vi "Compute Image ROI Statistics.vi"(6 "ROI Characteristics Selection":T1={"Area (pixels)"=TRUE, "% of Image"=TRUE, "Total Intensity"=TRUE, "Mean Intensity"=TRUE, "Median Intensity"=TRUE, "Mode Intensity"=TRUE, "Intensity Standard Deviation"=TRUE, "Min Intensity"=TRUE, "Max Intensity"=TRUE, "Mean SNR"=TRUE, "Median SNR"=TRUE, "Mode SNR"=TRUE, "SNR Standard Deviation"=TRUE, "Max SNR"=TRUE, "Min SNR"=TRUE, "# Rejected Pixels (NaN, Inf)"=TRUE, "# Negative Pixels"=TRUE, "Long Axis Length"=FALSE, "Short Axis Length"=FALSE, "Aspect Ratio"=FALSE}, 8 "error in (no error)":errorcluster, 9 "ROIs":T3(array[cluster]), 10 "ROI Mask Refnum":T4, 11 "Image Refnum":T4) -> (0 "error out":errorcluster, 1 "ROI Characteristics String":string, 3 "ROI Characteristics":T2[](array[typedef]))   [LabVIEW 2021, in "Image.lvlib"]
doc: "<B>Image Refnum</B> is the image to be analyzed.\n\n<B>ROI Mask Refnum</B> is the image used to store the mask image corresponding to the ROI (same type as source image). If no image is provided, a temporary one is c reated (and destroyed after use).\n\n<B>ROI</B> is the ROI descriptor."
uses:
  Image.lvlib
  <vilib>/vision/Image Controls.llb/IMAQ Image.ctl
  Image ROI Statistics.ctl
  Image ROI Statistics Selection.ctl
  <vilib>/vision/NI_Vision_Development_Module.lvlib
  Error/Error.lvlib
  Variant/Variant.lvlib
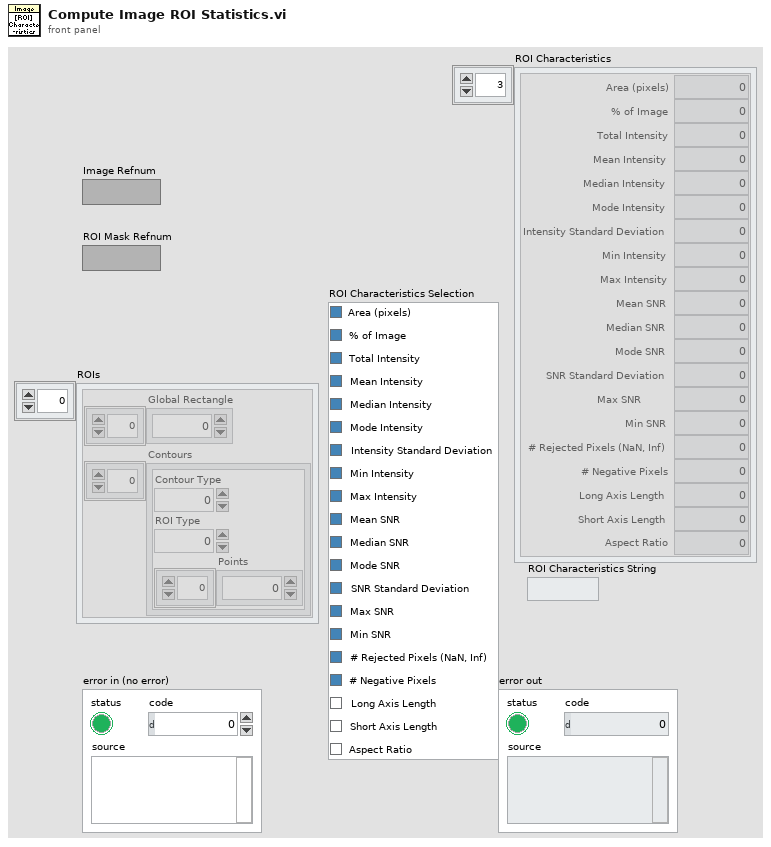
[diagram p1: front panel]
types:
  T1 = typedef "Image.lvlib/Image ROI Statistics Selection.ctl" = cluster{"Area (pixels)":bool, "% of Image":bool, "Total Intensity":bool, "Mean Intensity":bool, "Median Intensity":bool, "Mode Intensity":bool, "Intensity Standard Deviation":bool, "Min Intensity":bool, "Max Intensity":bool, "Mean SNR":bool, "Median SNR":bool, "Mode SNR":bool, "SNR Standard Deviation":bool, "Max SNR":bool, "Min SNR":bool, "# Rejected Pixels (NaN, Inf)":bool, "# Negative Pixels":bool, "Long Axis Length":bool, "Short Axis Length":bool, "Aspect Ratio":bool}
  T2 = typedef "Image.lvlib/Image ROI Statistics.ctl" = cluster{"Area (pixels)":dbl, "% of Image":dbl, "Total Intensity":dbl, "Mean Intensity":dbl, "Median Intensity":dbl, "Mode Intensity":dbl, "Intensity Standard Deviation":dbl, "Min Intensity":dbl, "Max Intensity":dbl, "Mean SNR":dbl, "Median SNR":dbl, "Mode SNR":dbl, "SNR Standard Deviation":dbl, "Max SNR":dbl, "Min SNR":dbl, "# Rejected Pixels (NaN, Inf)":dbl, "# Negative Pixels":dbl, "Long Axis Length":dbl, "Short Axis Length":dbl, "Aspect Ratio":dbl}
  T3 = cluster{"Global Rectangle":i32[], "Contours":cluster{"Contour Type":u32, "ROI Type":u32, "Points":i32[]}[]}[]
  T4 = typedef "IMAQ Image.ctl" = refnum<image>
  T5 = typedef "Image Type" = u32
  T6 = cluster{"Global Rectangle":i32[], "Contours":cluster{"Contour Type":u32, "ROI Type":u32, "Points":i32[]}[]}
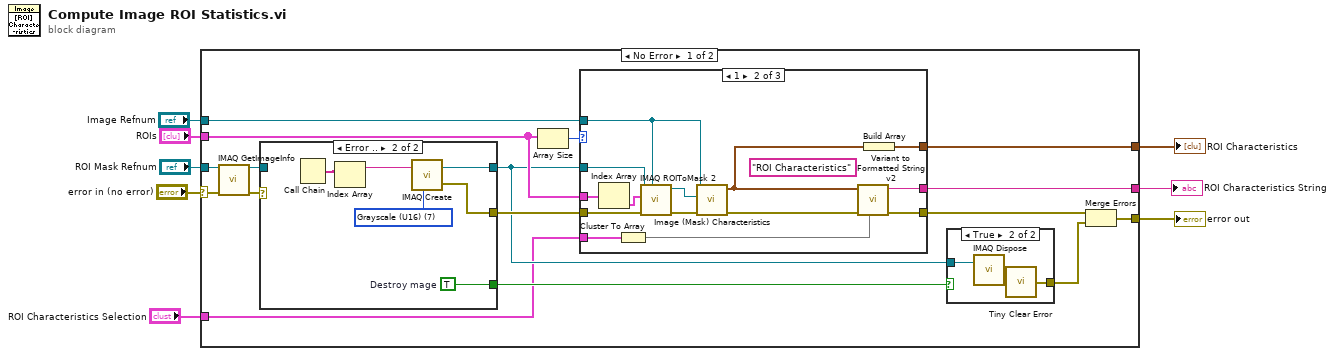
[diagram p0: block diagram]
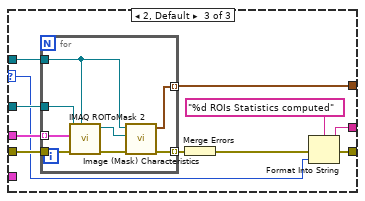
[diagram p4: hidden frame]
diagram:
  n1 = case shown="No Error" "error in (no error)" {
    selector: "error in (no error)" -> [w20 w69]
    tunnel: "Image Refnum" -> [w23 _]
    tunnel: [w22 _] -> w7
    tunnel: [w21 _] -> w6
    tunnel: [w11 w69] -> w5
    tunnel: "ROIs" -> [w16 _]
    tunnel: "ROI Mask Refnum" -> [w18 _]
    tunnel: "ROI Characteristics Selection" -> [w9 _]
    frame No Error {
      n2 = call "IMAQ GetImageInfo"("error in (no error)"=w20, "Image"=w18) -> ("error out"=w19:errorcluster)  [unwired: 2 in, 7 out]
      n3 = case shown="Error .." w19 {
        selector: w19 -> [w62 _]
        tunnel: [w62 w68] -> w17
        tunnel: w18 -> [w61 _]
        tunnel: [w61 w67] -> w13
        tunnel: [_ w63] -> w14
        frame No Error {
        }
        frame Error {
          w66 = T5 7 items=["Grayscale (U8)", "Grayscale (I16)", "Grayscale (SGL)", "Complex (CSG)", "RGB (U32)", "HSL (U32)", "RGB (U64)", "Grayscale (U16)"] ("Image Type")
          w63 = TRUE  # Destroy mage
          n4 = Call Chain() -> (call chain=w65:string[])
          n5 = Index Array(array=w65) -> (element=w64:string)  [unwired: 1 in]
          n6 = call "IMAQ Create"("Image Name"=w64, "Image Type"=w66) -> ("New Image"=w67:T4, "error out"=w68:errorcluster)  [unwired: 3 in]
        }
      }
      n7 = Array Size(array=w16) -> (size(s)=w15:i32)
      n8 = case shown="1" w15 {
        selector: w15 -> [_ _ w42]
        tunnel: w23 -> [_ w41 w52]
        tunnel: [_ w30 w51] -> w22
        tunnel: [_ w39 w44] -> w21
        tunnel: [w27 w38 w45] -> w10
        tunnel: w13 -> [_ w31 w49]
        tunnel: w17 -> [w27 w35 w50]
        tunnel: w16 -> [_ w34 w47]
        tunnel: w9 -> [_ w29 _]
        frame 0 {
        }
        frame 1 {
          (unwired) "ROI Characteristics" ("Label")
          n9 = Index Array(array=w34) -> (element=w33:T6)  [unwired: 1 in]
          n10 = Cluster To Array(cluster=w29) -> (array=w28:bool[])
          n11 = call "IMAQ ROIToMask 2"("Image Model"=w41, "error in (no error)"=w35, "ROI Descriptor"=w33, "Image"=w31) -> ("error out"=w37:errorcluster, "Image Out"=w36:T4)  [unwired: 5 in, 1 out]
          n12 = call "Image (Mask) Characteristics.vi"("error in (no error)"=w37, "Image Mask Refnum"=w36, "Image Refnum"=w41) -> ("error out"=w32:errorcluster, "Mask ROI Statistics"=w40:T2)  [unwired: 6 in, 1 out]
          n13 = call "Variant to Formatted String v2.vi"("Tokens to keep (all)"=w28, "error in (no error)"=w32, "Anything"=w40) -> ("error out"=w38:errorcluster, "String"=w39:string)  [unwired: 7 in]
          n14 = Build Array(w40) -> (w30:T2[])
        }
        frame 2, Default {
          n15 = for {
            tunnel: w52 -> [w54]
            tunnel: [w60] -> w51 mode=indexing
            tunnel: w49 -> [w56]
            tunnel: w50 -> [w57]
            tunnel: [w55] -> w48 mode=indexing
            tunnel: w47 -> [w53] mode=indexing
            n16 = call "IMAQ ROIToMask 2"("Image Model"=w54, "error in (no error)"=w57, "ROI Descriptor"=w53, "Image"=w56) -> ("error out"=w59:errorcluster, "Image Out"=w58:T4)  [unwired: 5 in, 1 out]
            n17 = call "Image (Mask) Characteristics.vi"("error in (no error)"=w59, "Image Mask Refnum"=w58, "Image Refnum"=w54) -> ("error out"=w55:errorcluster, "Mask ROI Statistics"=w60:T2)  [unwired: 6 in, 1 out]
          }
          n18 = Merge Errors(w48) -> (w46:errorcluster)
          n19 = Format Into String(format string="%d ROIs Statistics computed", error in=w46, w42) -> (resulting string=w44:string, error out=w45:errorcluster)  [unwired: 1 in]
        }
      }
      n20 = case shown="True" w14 {
        tunnel: w13 -> [_ w25]
        tunnel: [_ w24] -> w12
        frame False {
        }
        frame True {
          n21 = call "IMAQ Dispose"("Image"=w25) -> ("error out"=w26:errorcluster)  [unwired: 5 in]
          n22 = call "Tiny Clear Error.vi"("Error In"=w26) -> ("no Error Out"=w24:errorcluster)  [unwired: 8 in]
        }
      }
      n23 = Merge Errors(w10, w12) -> (w11:errorcluster)
    }
    frame Error {
    }
  }
  "ROI Characteristics String" <- w6
  "error out" <- w5
  "ROI Characteristics" <- w7
